vi "New Round.vi"(11 "Team in":refnum<class "Team.lvclass">) -> (3 "Team out":refnum<class "Team.lvclass">)   [LabVIEW 2020, in "SquareBattle.lvlib" / "Team.lvclass"]
doc: "This VI is called once at the beginning of each new round. This can be used to do global map updates, coordinated plans for all active squares, or nothing at all!"
uses:
  Team.lvclass
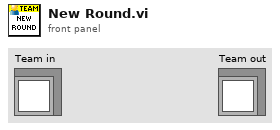
[diagram p1: front panel]
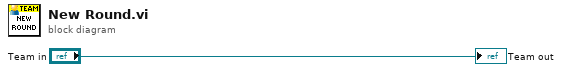
[diagram p0: block diagram]
diagram:
  "Team out" <- "Team in"
